vi "TTA_MATLAB_Perform_Siggen_Amp_CAL.vi"(0 "IF Frequency (MHz)":dbl, 1 "MXG VISA Resource In":refnum<visa-resource-name>, 2 "EXA VISA Resource":refnum<visa-resource-name>, 5 "IF Index":i32, 7 "Test":string(combo), 9 "Amp CAL Criteria Cluster":T1, 11 "error in":errorcluster) -> (4 "ACP Power":dbl, 6 "SigGen Power":dbl, 12 "MXG VISA Resource Out":refnum<visa-resource-name>, 13 "EXA VISA Resource Out":refnum<visa-resource-name>, 15 "error out":errorcluster)   [LabVIEW 2016]
uses:
  TTA_Globals/TTA_Global_Complete_Settings.vi
panel:
  in  "PALLinearization Values":T2
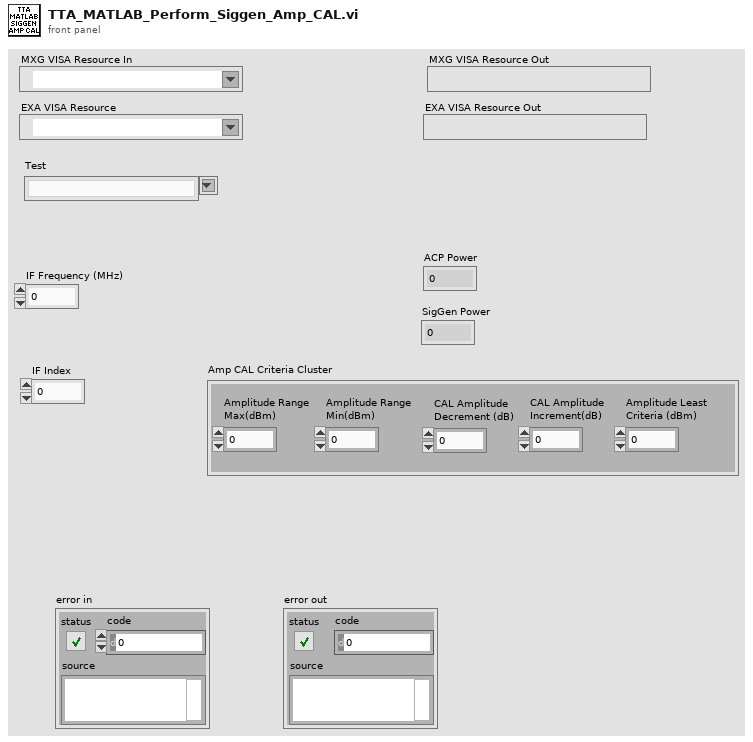
[diagram p1: front panel]
types:
  T1 = cluster{"Amplitude Range\nMax(dBm)":dbl, "Amplitude Range\nMin(dBm)":dbl, "CAL Amplitude\nDecrement (dB)":dbl, "CAL Amplitude\nIncrement(dB)":dbl, "Amplitude Least\nCriteria (dBm)":dbl}
  T2 = cluster{"Tx IF Offsets":dbl[], "ACPR Filename":string, "Sampling Rate":dbl, "TxIF_Freq":dbl, "Power (dBm)":dbl, "IF Frequency Sweep (MHz)":dbl[], "BDSFreq":dbl, "Amplitude Range\nMax(dBm)":dbl, "Amplitude Range\nMin(dBm)":dbl, "CAL Amplitude\nIncrement(dB)":dbl, "CAL Amplitude\nDecrement (dB)":dbl, "Amplitude Least\nCriteria (dBm)":dbl}
  T3 = typedef "TTA_Control_Complete_Settings_Cluster.ctl" = cluster{"Brief Cluster":cluster{"STM Firmware File":string, "STM Firmware Address":string, "Required SW Version":string, "Template Used":string}, "Instrument Setting Cluster":cluster{"BDSFreq":dbl, "BDS Amp":dbl, "TxRFCal_Freq":dbl, "TxRFCal_Amp":dbl, "RxRFCal_Freq":dbl, "RxRFCal_Freq":dbl, "TxIF_Freq":dbl, "TxIF_Amp":dbl, "Tx_Output_Power_Signal_Freq":dbl, "Tx_ACPR_Signal_Freq":dbl, "Rx_RF_Freq":dbl, "Rx_RF_Amp":dbl, "Rx_Output_Power_Signal_Freq":dbl, "Rx_Output_Power_Sense_Freq":dbl}, "PAL Calibration\nInputs Cluster":cluster{"Amplitude Range\nMax(dBm)":dbl, "Amplitude Range\nMin(dBm)":dbl, "Amplitude Least\nCriteria (dBm)":dbl, "Frequency 1":dbl, "Frequency 2":dbl, "Frequency 3":dbl, "CAL Amplitude\nDecrement (dB)":dbl, "CAL Amplitude\nIncrement(dB)":dbl, "DownloadFile":string}, "TxOffset Cal Cluster":cluster{"Tx1 Offset (dB)":dbl, "Tx2 Offset (dB)":dbl, "Tx3 Offset (dB)":dbl, "Tx4 Offset (dB)":dbl, "Total RF Tx Loss (dB)":dbl}, "RxOffset Cal Cluster":cluster{"Rx1 Offset (dB)":dbl, "Rx2 Offset (dB)":dbl, "Rx3 Offset (dB)":dbl, "Rx4 Offset (dB)":dbl, "Total RF Rx Loss (dB)":dbl}, "TX Output Power Settings Cluster":cluster{"Frequency Sweep (MHz)":dbl[], "Sig Gen \nPower (dBm)":dbl, "Span (kHz)":dbl, "RBW (Hz)":dbl, "Ref Level (dBm)":dbl, "Low Power \nLimit":dbl, "High Power \nLimit":dbl, "DigAtt Max":dbl, "DigAtt Min":dbl}, "Tx ACPR Settings Cluster":cluster{"ACPR Filename":string, "Sampling Rate":dbl, "Power (dBm)":dbl, "IF Frequency Sweep (MHz)":dbl[], "State Name":string, "Mechanical\nAttenuation":dbl, "RefLevel Offset":dbl, "Amplitude Range\nMax (dBm)":dbl, "Amplitude Range\nMin (dBm)":dbl, "Cal Amp \nIncrement (dB)":dbl, "Cal Amp\nDecrement (dB)":dbl}, "Power Cal Cluster":cluster{"Power List (dBm)":dbl[], "Frequency (MHz)":dbl[], "Cal Decrement (dB)":dbl, "Cal Increment (dB)":dbl}, "Rx Received Power Settings Cluster":cluster{"Frequency Sweep (MHz)":dbl[], "Power (dBm)":dbl, "Span (kHz)":dbl, "RBW (Hz)":dbl, "Ref Level":dbl, "Low Power \nLimit (dBm)":dbl, "High Power\nLimit (dBm)":dbl}, "Tx Output Power Criteria Cluster":cluster{"CH1-TX1 \nMin":dbl, "CH1-TX1\nMax":dbl, "CH1-TXx3\nMin ":dbl, "CH1-TXx3\nMax":dbl, "CH2-TX1\nMin":dbl, "CH2-TX1\nMax":dbl, "CH2-TXx3\nMin":dbl, "CH2-TXx3\nMax":dbl}, "Tx ACPR Criteria Cluster":cluster{"Min Inband":dbl, "Max Close Outband":dbl, "Max Far Outband":dbl}, "Rx Output Power Criteria Cluster":cluster{"CH1-RX1 \nMin":dbl, "CH1-RX1 \nMax":dbl, "CH1-RXx3 \nMin":dbl, "CH1-RXx3\nMax":dbl, "CH2-RX1\nMin":dbl, "CH2-RX1\nMax":dbl, "CH2-RXx3\nMin":dbl, "CH2-RXx3\nMax":dbl}}
  T4 = cluster{"BDSFreq":dbl, "BDS Amp":dbl, "TxRFCal_Freq":dbl, "TxRFCal_Amp":dbl, "RxRFCal_Freq":dbl, "RxRFCal_Freq":dbl, "TxIF_Freq":dbl, "TxIF_Amp":dbl, "Tx_Output_Power_Signal_Freq":dbl, "Tx_ACPR_Signal_Freq":dbl, "Rx_RF_Freq":dbl, "Rx_RF_Amp":dbl, "Rx_Output_Power_Signal_Freq":dbl, "Rx_Output_Power_Sense_Freq":dbl}
  T5 = cluster{"Tx1 Offset (dB)":dbl, "Tx2 Offset (dB)":dbl, "Tx3 Offset (dB)":dbl, "Tx4 Offset (dB)":dbl, "Total RF Tx Loss (dB)":dbl}
  T6 = cluster{"ACPR Filename":string, "Sampling Rate":dbl, "Power (dBm)":dbl, "IF Frequency Sweep (MHz)":dbl[], "State Name":string, "Mechanical\nAttenuation":dbl, "RefLevel Offset":dbl, "Amplitude Range\nMax (dBm)":dbl, "Amplitude Range\nMin (dBm)":dbl, "Cal Amp \nIncrement (dB)":dbl, "Cal Amp\nDecrement (dB)":dbl}
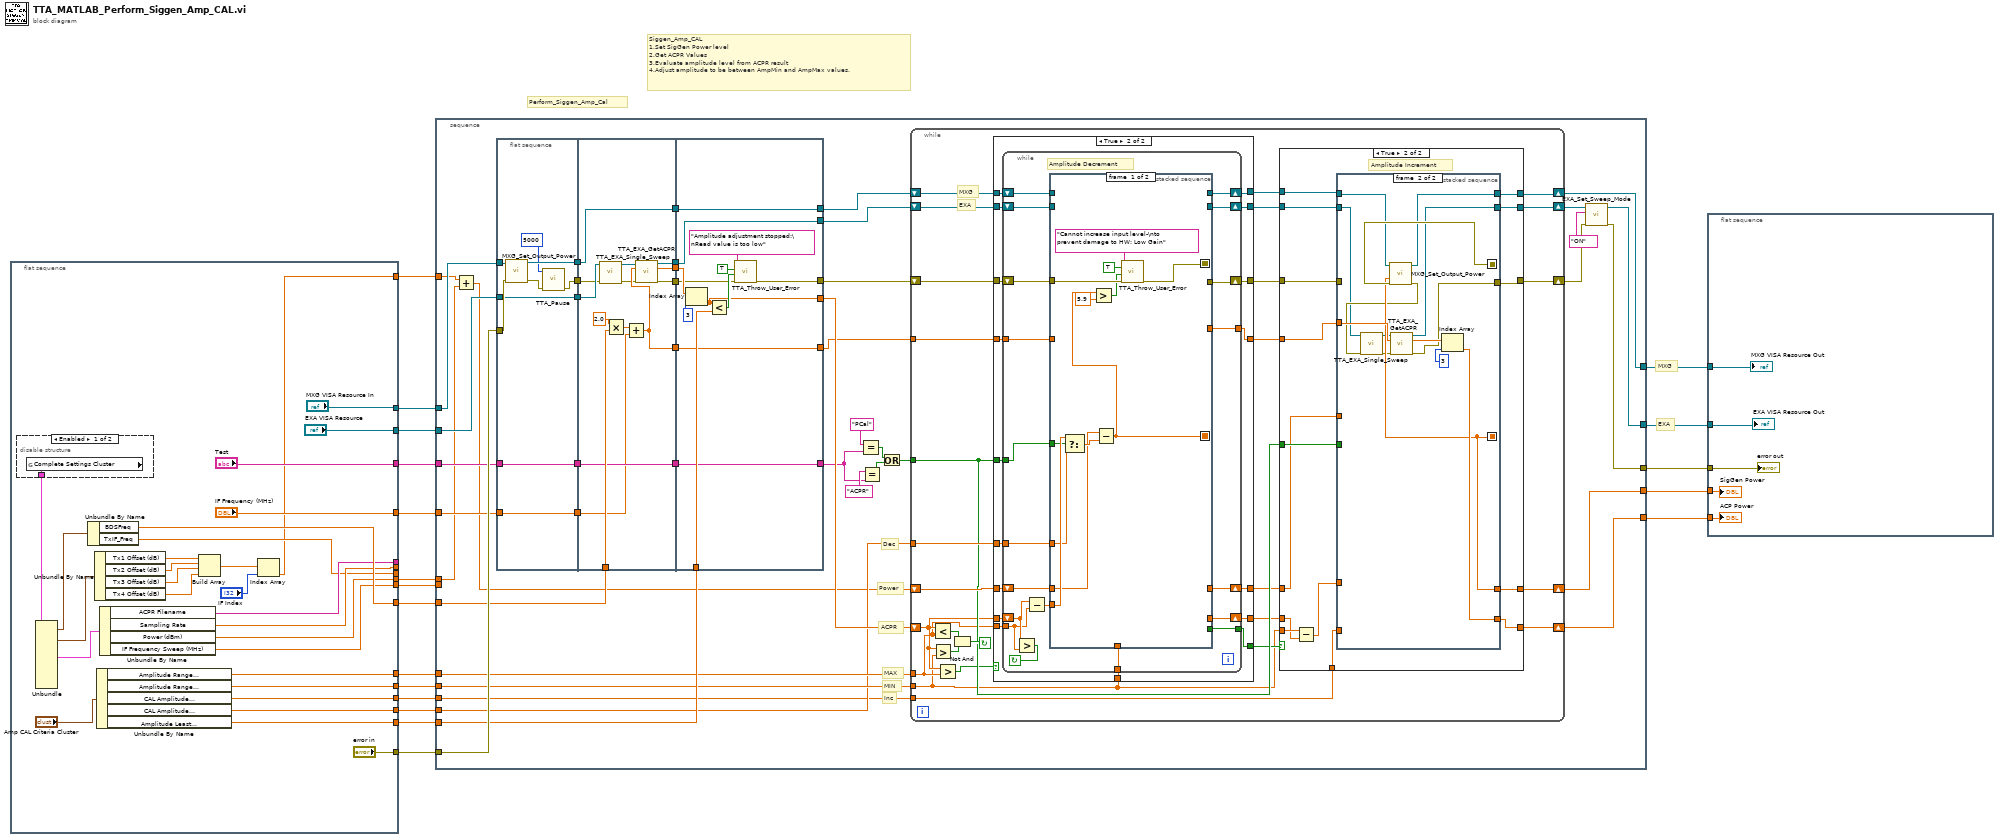
[diagram p0: block diagram]
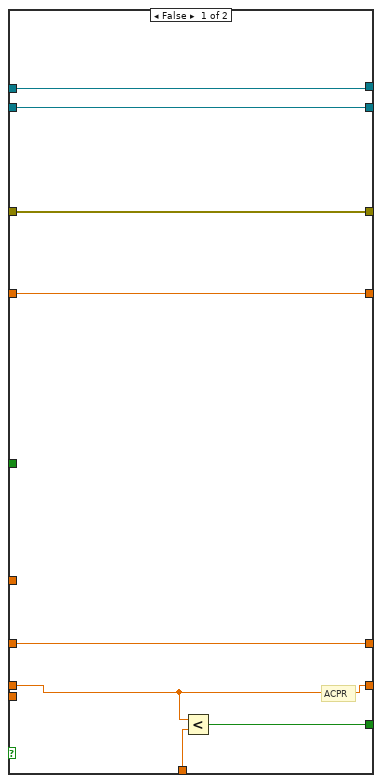
[diagram p2: hidden frame]
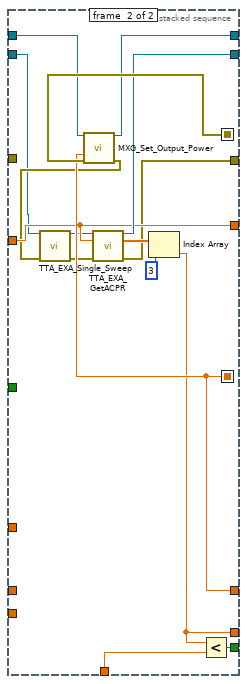
[diagram p3: hidden frame]
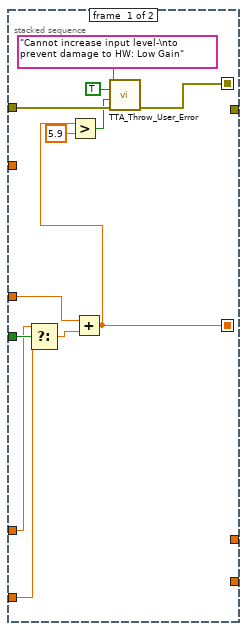
[diagram p5: hidden frame]
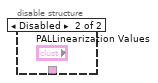
[diagram p6: hidden frame]
diagram:
  # "Siggen_Amp_CAL\n1.Set SigGen Power level\n2.Get ACPR Values \n3.Evaluate amplitude level from ACPR result\n4.Adjust amplitude to be between AmpMin and AmpMax values."
  # "EXA"
  # "MXG"
  # "Perform_Siggen_Amp_Cal"
  n1 = flat-sequence {
    tunnel: ["error in"] -> w19
    tunnel: ["MXG VISA Resource In"] -> w18
    tunnel: ["EXA VISA Resource"] -> w17
    tunnel: [w31] -> _
    tunnel: [w34] -> _
    tunnel: [w35] -> _
    tunnel: [w33] -> w2
    tunnel: [w32] -> w12
    tunnel: [w40] -> w5
    tunnel: [w30] -> w11
    tunnel: [w29] -> w10
    tunnel: [w28] -> w9
    tunnel: [w27] -> w8
    tunnel: [w26] -> w7
    tunnel: ["Test"] -> w4
    tunnel: ["IF Frequency (MHz)"] -> w6
    tunnel: [w21] -> w1
    frame #0 {
      n2 = disable-structure shown="Enabled" {
        disable-tunnel: [w48 _] -> w44
        frame Enabled {
          n3 = global read "TTA_Global_Complete_Settings.vi" "Complete Settings Cluster"() -> (w48:T3)
        }
        frame Disabled {
        }
      }
      n4 = Unbundle(w44) -> ("Instrument Setting Cluster"=w43:T4, "TxOffset Cal Cluster"=w42:T5, "Tx ACPR Settings Cluster"=w41:T6)  [unwired: 9 out]
      n5 = Unbundle By Name(w43) -> ("BDSFreq"=w40:dbl, "TxIF_Freq"=w31:dbl)
      n6 = Unbundle By Name(w42) -> ("Tx1 Offset (dB)"=w39:dbl, "Tx2 Offset (dB)"=w38:dbl, "Tx3 Offset (dB)"=w37:dbl, "Tx4 Offset (dB)"=w36:dbl)
      n7 = Unbundle By Name("Amp CAL Criteria Cluster") -> ("Amplitude Range\nMax(dBm)"=w30:dbl, "Amplitude Range\nMin(dBm)"=w29:dbl, "CAL Amplitude\nIncrement(dB)"=w28:dbl, "CAL Amplitude\nDecrement (dB)"=w27:dbl, "Amplitude Least\nCriteria (dBm)"=w26:dbl)
      n8 = Unbundle By Name(w41) -> ("ACPR Filename"=w35:string, "Sampling Rate"=w34:dbl, "Power (dBm)"=w33:dbl, "IF Frequency Sweep (MHz)"=w32:dbl[])
      n9 = Build Array(w39, w38, w37, w36) -> (w23:dbl[])
      n10 = Index Array(array=w23, index="IF Index") -> (element=w21:dbl)
    }
  }
  n11 = stacked-sequence {
    tunnel: w19 -> [w92]
    tunnel: w18 -> [w91]
    tunnel: w17 -> [w88]
    tunnel: [w52] -> w16
    tunnel: [w61] -> w15
    tunnel: [w60] -> w14
    tunnel: [w49] -> w13
    tunnel: w12 -> [_]
    tunnel: w11 -> [w76]
    tunnel: w10 -> [w75]
    tunnel: w9 -> [w62]
    tunnel: w8 -> [w71]
    tunnel: w7 -> [w82]
    tunnel: w2 -> [w55]
    tunnel: w6 -> [w58]
    tunnel: w5 -> [w86]
    tunnel: w4 -> [w74]
    tunnel: [w59] -> w3
    tunnel: w1 -> [w56]
    frame #0 {
      # "Inc"
      # "Dec"
      # "Power"
      # "MIN"
      # "MAX"
      # "ACPR"
      n12 = Add(x=w56, y=w55) -> (x+y=w54:dbl)
      n13 = flat-sequence {
        tunnel: w92 -> [w245]
        tunnel: w91 -> [w246]
        tunnel: [w239] -> w90
        tunnel: [w244] -> w89
        tunnel: w88 -> [w243]
        tunnel: [w243] -> w87
        tunnel: w74 -> [w242]
        tunnel: [w242] -> w73
        tunnel: w58 -> [w241]
        tunnel: [w241] -> w57
        tunnel: w90 -> [w248]
        tunnel: w89 -> [w254]
        tunnel: w87 -> [w249]
        tunnel: w86 -> [w260]
        tunnel: [w257] -> w85
        tunnel: [w256] -> w84
        tunnel: [w255] -> w83
        tunnel: [w254] -> w81
        tunnel: w73 -> [w253]
        tunnel: [w253] -> w72
        tunnel: [w252] -> w70
        tunnel: w57 -> [w251]
        tunnel: w85 -> [w265]
        tunnel: w84 -> [w269]
        tunnel: w83 -> [w273]
        tunnel: w82 -> [w271]
        tunnel: w81 -> [w266]
        tunnel: [w266] -> w80
        tunnel: [w265] -> w79
        tunnel: [w264] -> w78
        tunnel: [w263] -> w77
        tunnel: w72 -> [w262]
        tunnel: [w262] -> w64
        tunnel: w70 -> [w261]
        tunnel: [w261] -> w69
        frame #0 {
          n14 = call "MXG_Set_Output_Power.vi"("VISA resource name"=w246, "error in"=w245) -> ("VISA resource name"=w244:refnum<visa-resource-name>, "error out"=w240:errorcluster)  [unwired: 12 in]
          n15 = call "TTA_Pause.vi"("error in"=w240, "Pause (ms)"=u32 5000) -> ("error out"=w239:errorcluster)  [unwired: 9 in]
        }
        frame #1 {
          n16 = call "TTA_EXA_Single_Sweep.vi"("VISA resource In"=w249, "error in"=w248) -> ("VISA resource Out"=w247:refnum<visa-resource-name>, "error out"=w250:errorcluster)  [unwired: 11 in, 1 out]
          n17 = Multiply(x=2.0, y=w260) -> (x*y=w258:dbl)
          n18 = Add(x=w258, y=w251) -> (x+y=w252:dbl)
          n19 = call "TTA_EXA_GetACPR.vi"("VISA resource In"=w247, "Frequency (MHz)"=w252, "error in"=w250) -> ("VISA resource Out"=w257:refnum<visa-resource-name>, "ACP Values"=w255:dbl[], "error out"=w256:errorcluster)  [unwired: 9 in, 1 out]
        }
        frame #2 {
          n20 = Index Array(array=w273, index=3) -> (element=w263:dbl)
          n21 = Less?(x=w263, y=w271) -> (x < y?=w270:bool)
          n22 = call "TTA_Throw_User_Error.vi"("error in"=w269, "Error?"=w270, "Stop Execution on Fail"=TRUE, "Error Message"="Amplitude adjustment stopped:\nRead value is too low") -> ("error out"=w264:errorcluster)  [unwired: 7 in]
        }
      }
      n23 = Equal?(x="PCal", y=w64) -> (x = y?=w68:bool)
      n24 = Equal?(x="ACPR", y=w64) -> (x = y?=w67:bool)
      n25 = Or(x=w68, y=w67) -> (x .or. y?=w63:bool)
      n26 = while {
        shift-right: [w97] -> w50
        shift-left: w78 -> [w117]
        shift-right: [w101] -> w60
        shift-left: w77 -> [w109]
        tunnel: w76 -> [w108]
        tunnel: w75 -> [w94]
        shift-right: [w93] -> w59
        shift-left: w54 -> [w112]
        tunnel: w71 -> [w113]
        tunnel: w69 -> [w111]
        tunnel: w63 -> [w110]
        shift-right: [w99] -> w61
        shift-left: w80 -> [w119]
        shift-right: [w98] -> w53
        shift-left: w79 -> [w118]
        tunnel: w62 -> [w95]
        stop <- w114 continue-if-true
        # "EXA"
        # "MXG"
        n27 = Less?(x=w109, y=w108) -> (x < y?=w116:bool)
        n28 = Greater?(x=w109, y=w94) -> (0:w115:bool)
        n29 = Greater?(x=w109, y=w108) -> (0:w107:bool)
        n30 = Not And(1:w115, 2:w116) -> (0:w114:bool)
        n31 = case shown="True" w107 {
          tunnel: w119 -> [w127 w144]
          tunnel: w118 -> [w126 w143]
          tunnel: w117 -> [w125 w142]
          tunnel: w109 -> [w122 w141]
          tunnel: w108 -> [_ w140]
          tunnel: w113 -> [_ w139]
          tunnel: w112 -> [w123 w138]
          tunnel: w111 -> [w124 w137]
          tunnel: w110 -> [_ w136]
          tunnel: [w127 w135] -> w106
          tunnel: [w126 w134] -> w105
          tunnel: [w125 w133] -> w104
          tunnel: [w122 w132] -> w102
          tunnel: [w124 w131] -> w103
          tunnel: [w123 w130] -> w100
          tunnel: w94 -> [w121 w129]
          tunnel: [w120 w128] -> w96
          frame False {
            # "ACPR"
            n32 = Less?(x=w122, y=w121) -> (x < y?=w120:bool)
          }
          frame True {
            n33 = while {
              shift-right: [w153] -> w135
              shift-left: w144 -> [w163]
              shift-right: [w152] -> w134
              shift-left: w143 -> [w162]
              shift-right: [w149] -> w133
              shift-left: w142 -> [w161]
              shift-right: [w151] -> w132
              shift-left: w141 -> [w159]
              tunnel: w140 -> [w158]
              tunnel: w139 -> [w156]
              shift-right: [w150] -> w130
              shift-left: w138 -> [w155]
              tunnel: w137 -> [w154]
              tunnel: w136 -> [w148]
              tunnel: [w147] -> w131
              tunnel: w129 -> [w146]
              tunnel: [w145] -> w128
              stop <- w160 continue-if-true
              # "Amplitude Decrement"
              n34 = Greater?(x=w159, y=w158) -> (0:w160:bool)
              n35 = Subtract(x=w159, y=w158) -> (x-y=w157:dbl)
              n36 = stacked-sequence {
                seq-local: [w165 _] -> [_ w185]
                seq-local: [w166 _] -> [_ w191]
                tunnel: w163 -> [_ w190]
                tunnel: w162 -> [_ w177]
                tunnel: w161 -> [w171 _]
                tunnel: w157 -> [w175 _]
                tunnel: w156 -> [w174 _]
                tunnel: w155 -> [w172 _]
                tunnel: w154 -> [_ w184]
                tunnel: [_ w187] -> w153
                tunnel: [_ w186] -> w152
                tunnel: [_ w183] -> w151
                tunnel: [_ w185] -> w150
                tunnel: [_ w180] -> w149
                tunnel: w148 -> [w164 _]
                tunnel: [_ w184] -> w147
                tunnel: w146 -> [_ w182]
                tunnel: [_ w181] -> w145
                frame #0 {
                  n37 = Select(t=w175, s=w164, f=w174) -> (s? t:f=w173:dbl)
                  n38 = Subtract(x=w172, y=w173) -> (x-y=w165:dbl)
                  n39 = Greater?(x=w165, y=5.9) -> (0:w168:bool)
                  n40 = call "TTA_Throw_User_Error.vi"("error in"=w171, "Error?"=w168, "Stop Execution on Fail"=TRUE, "Error Message"="Cannot increase input level-\nto prevent damage to HW: Low Gain") -> ("error out"=w166:errorcluster)  [unwired: 7 in]
                }
                frame #1 {
                  n41 = call "MXG_Set_Output_Power.vi"("VISA resource name"=w190, "Output Power\nLevel (dBm)"=w185, "error in"=w191) -> ("VISA resource name"=w187:refnum<visa-resource-name>, "error out"=w179:errorcluster)  [unwired: 11 in]
                  n42 = call "TTA_EXA_Single_Sweep.vi"("VISA resource In"=w177, "error in"=w179) -> ("VISA resource Out"=w176:refnum<visa-resource-name>, "error out"=w178:errorcluster)  [unwired: 11 in, 1 out]
                  n43 = call "TTA_EXA_GetACPR.vi"("VISA resource In"=w176, "Frequency (MHz)"=w184, "error in"=w178) -> ("VISA resource Out"=w186:refnum<visa-resource-name>, "ACP Values"=w188:dbl[], "error out"=w180:errorcluster)  [unwired: 9 in, 1 out]
                  n44 = Index Array(array=w188, index=3) -> (element=w183:dbl)
                  n45 = Less?(x=w183, y=w182) -> (x < y?=w181:bool)
                }
              }
            }
          }
        }
        n46 = case shown="True" w96 {
          tunnel: w110 -> [_ w211]
          tunnel: w106 -> [w195 w210]
          tunnel: w105 -> [w194 w209]
          tunnel: w104 -> [w193 w208]
          tunnel: w103 -> [_ w207]
          tunnel: w102 -> [w196 w199]
          tunnel: [w196 w205] -> w101
          tunnel: w100 -> [w192 w206]
          tunnel: [w195 w204] -> w99
          tunnel: [w194 w203] -> w98
          tunnel: [w193 w202] -> w97
          tunnel: w95 -> [_ w201]
          tunnel: w94 -> [_ w200]
          tunnel: [w192 w197] -> w93
          frame False {
          }
          frame True {
            # "Amplitude Increment"
            n47 = Subtract(x=w200, y=w199) -> (x-y=w198:dbl)
            n48 = stacked-sequence {
              seq-local: [w212 _] -> [_ w229]
              seq-local: [w213 _] -> [_ w237]
              tunnel: w210 -> [_ w236]
              tunnel: w209 -> [_ w224]
              tunnel: w208 -> [w218 _]
              tunnel: w198 -> [w222 _]
              tunnel: w211 -> [w223 _]
              tunnel: w201 -> [w221 _]
              tunnel: w206 -> [w219 _]
              tunnel: w207 -> [_ w235]
              tunnel: [_ w232] -> w204
              tunnel: [_ w231] -> w203
              tunnel: [_ w230] -> w205
              tunnel: [_ w229] -> w197
              tunnel: [_ w228] -> w202
              frame #0 {
                n49 = Select(t=w222, s=w223, f=w221) -> (s? t:f=w220:dbl)
                n50 = Add(x=w219, y=w220) -> (x+y=w212:dbl)
                n51 = Greater?(x=w212, y=5.9) -> (0:w215:bool)
                n52 = call "TTA_Throw_User_Error.vi"("error in"=w218, "Error?"=w215, "Stop Execution on Fail"=TRUE, "Error Message"="Cannot increase input level-\nto prevent damage to HW: Low Gain") -> ("error out"=w213:errorcluster)  [unwired: 7 in]
              }
              frame #1 {
                n53 = call "MXG_Set_Output_Power.vi"("VISA resource name"=w236, "Output Power\nLevel (dBm)"=w229, "error in"=w237) -> ("VISA resource name"=w232:refnum<visa-resource-name>, "error out"=w225:errorcluster)  [unwired: 11 in]
                n54 = call "TTA_EXA_Single_Sweep.vi"("VISA resource In"=w224, "error in"=w225) -> ("VISA resource Out"=w227:refnum<visa-resource-name>, "error out"=w226:errorcluster)  [unwired: 11 in, 1 out]
                n55 = call "TTA_EXA_GetACPR.vi"("VISA resource In"=w227, "Frequency (MHz)"=w235, "error in"=w226) -> ("VISA resource Out"=w231:refnum<visa-resource-name>, "ACP Values"=w233:dbl[], "error out"=w228:errorcluster)  [unwired: 9 in, 1 out]
                n56 = Index Array(array=w233, index=3) -> (element=w230:dbl)
              }
            }
          }
        }
      }
      n57 = call "EXA_Set_Sweep_Mode.vi"("error in"=w50, "Continous"="ON", "VISA resource name"=w53) -> ("error out"=w49:errorcluster, "VISA resource name"=w52:refnum<visa-resource-name>)  [unwired: 7 in]
    }
  }
  n58 = flat-sequence {
    tunnel: w16 -> [w278]
    tunnel: w15 -> [w277]
    tunnel: w14 -> [w276]
    tunnel: w13 -> [w275]
    tunnel: w3 -> [w274]
    frame #0 {
      "error out" <- w275
      "MXG VISA Resource Out" <- w277
      "EXA VISA Resource Out" <- w278
      "ACP Power" <- w276
      "SigGen Power" <- w274
    }
  }
